vi "Set_Parameter_Instrument (Json).vi"(8 "error in (no error)":errorcluster caption="entrée d'erreur (pas d'erreur)", 10 "Parameter (Json)":string, 11 "Pattern_Matching en entrée":refnum<class "Pattern_Matching.lvclass">) -> (0 "error out":errorcluster caption="sortie d'erreur", 3 "Pattern_Matching en sortie":refnum<class "Pattern_Matching.lvclass">)   [LabVIEW 2020, in "Library Test.lvlib" / "Pattern_Matching.lvclass"]
uses:
  Pattern_Matching.lvclass
  C:/Users/ngarcin/OneDrive - Altyor/Standard TB/Class/Test/Test (Default)/Test (Default).lvclass
  Commun VI/TypeDef/Commande Pattern_Matching/Commande Parameter.ctl
  Camera/Class Camera Pattern Matching (Default)/Class Pattern Matching (Default).lvclass
  JSON API/JSON Value/Set from JSON string.vi
  JSON API/Variant JSON/Variant to JSON.vi
  JSON API/JSON Value/Get Item by name array.vi
  Test_Wtih_Instr/Test_With_Inst.lvclass
  Instrument/Instrument (Default)/Class Instrument (Default).lvclass
  JSON API/JSON Value/JSON Value.lvclass
  Pattern_Matching.lvclass/Pattern_Matching.ctl
  JSON API/Variant JSON/Variant JSON.lvlib
  JSON API/Get Polymorphic/JSON GetSet.lvlib
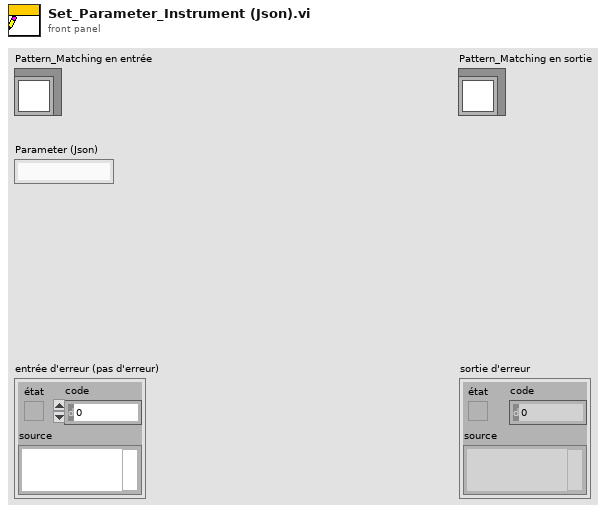
[diagram p1: front panel]
types:
  T1 = cluster{"Number Prog":string, "Test Number":u16, "Timeout":u16}
  T2 = typedef "Commande Parameter.ctl" = cluster{"Device_Addr":string, "Port":string, "Number Prog":string, "Test Number":u16, "Timeout":u16, "Library Pattern Matching":refnum<class "Class Pattern Matching (Default).lvclass">}
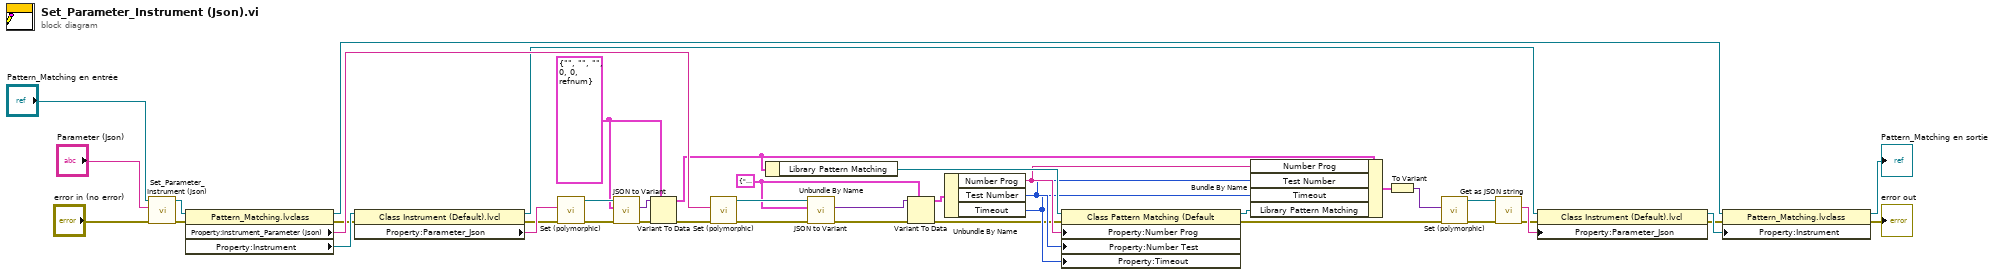
[diagram p0: block diagram]
diagram:
  w9 = T1 {"Number Prog"="", "Test Number"=0, "Timeout"=0} ("Parameter")
  w12 = T2 {"Device_Addr"="", "Port"="", "Number Prog"="", "Test Number"=0, "Timeout"=0, "Library Pattern Matching"=refnum} ("Parameter")
  n1 = call-parent "Set_Parameter_Instrument (Json).vi"("error in (no error)"="error in (no error)", "Parameter (Json)"="Parameter (Json)", "Test (Default) en entrée"="Pattern_Matching en entrée") -> ("error out"=w18:errorcluster, "Test (Default) en sortie"=w17:refnum<class "Pattern_Matching.lvclass">)  [unwired: 7 in]
  n2 = property class="Pattern_Matching.lvclass"(reference=w17, error in=w18) -> (reference out=w22:refnum<class "Pattern_Matching.lvclass">, error out=w13:errorcluster, "Property:Instrument_Parameter (Json)"=w24:string, "Property:Instrument"=w25:refnum<class "Class Instrument (Default).lvclass">)
  n3 = property class="Class Instrument (Default).lvcl"(reference=w25, error in=w13) -> (reference out=w21:refnum<class "Class Instrument (Default).lvclass">, error out=w29:errorcluster, "Property:Parameter_Json"=w31:string)
  n4 = call-poly "Set (polymorphic).vi"("error in (no error)"=w29, "JSON stream"=w31) -> ("error out"=w33:errorcluster, "JSON Value out"=w35:refnum<class "JSON Value.lvclass">)  [unwired: 7 in, 1 out]
  n5 = call "JSON to Variant.vi"("error in (no error)"=w33, "Variant (Data Type)"=w12, "JSON Value"=w35) -> ("error out"=w34:errorcluster, "Variant out"=w32:variant)  [unwired: 7 in]
  n6 = Variant To Data(error in=w34, type=w12, Variant=w32) -> (data=w8:T2, error out=w30:errorcluster)
  n7 = call-poly "Set (polymorphic).vi"("error in (no error)"=w30, "JSON stream"=w24) -> ("error out"=w38:errorcluster, "JSON Value out"=w36:refnum<class "JSON Value.lvclass">)  [unwired: 7 in, 1 out]
  n8 = Unbundle By Name(w8) -> ("Library Pattern Matching"=w7:refnum<class "Class Pattern Matching (Default).lvclass">)
  n9 = call "JSON to Variant.vi"("error in (no error)"=w38, "Variant (Data Type)"=w9, "JSON Value"=w36) -> ("error out"=w37:errorcluster, "Variant out"=w39:variant)  [unwired: 7 in]
  n10 = Variant To Data(error in=w37, type=w9, Variant=w39) -> (data=w19:T1, error out=w2:errorcluster)
  n11 = Unbundle By Name(w19) -> ("Number Prog"=w6:string, "Test Number"=w5:u16, "Timeout"=w4:u16)
  n12 = property class="Class Pattern Matching (Default"(reference=w7, error in=w2, "Property:Number Prog"=w6, "Property:Number Test"=w5, "Property:Timeout"=w4) -> (reference out=w3:refnum<class "Class Pattern Matching (Default).lvclass">, error out=w1:errorcluster)
  n13 = Bundle By Name(cluster=w8, "Number Prog"=w6, "Test Number"=w5, "Timeout"=w4, "Library Pattern Matching"=w3) -> (w20:T2)
  n14 = To Variant(anything=w20) -> (Variant=w27:variant)
  n15 = call-poly "Set (polymorphic).vi"("error in (no error)"=w1, "Variant"=w27) -> ("error out"=w16:errorcluster, "JSON Value out"=w28:refnum<class "JSON Value.lvclass">)  [unwired: 8 in]
  n16 = call "Get as JSON string.vi"("error in (no error)"=w16, "JSON Value in"=w28) -> ("error out"=w15:errorcluster, "<JSON>"=w26:string)  [unwired: 8 in]
  n17 = property class="Class Instrument (Default).lvcl"(reference=w21, error in=w15, "Property:Parameter_Json"=w26) -> (reference out=w23:refnum<class "Class Instrument (Default).lvclass">, error out=w14:errorcluster)
  n18 = property class="Pattern_Matching.lvclass"(reference=w22, error in=w14, "Property:Instrument"=w23) -> (reference out=→"Pattern_Matching en sortie":refnum<class "Pattern_Matching.lvclass">, error out=→"error out":errorcluster)
